vi "simulated camera.vi"(8 "error in (no error)":errorcluster) -> (0 "error out":errorcluster)   [LabVIEW 2018]
uses:
  Sim_Ixon_Ultra/Sim_Ixon_Ultra.lvclass
  C:/Users/Denis/Desktop/S4ACS/S4ACS/Sim_CCD/Sim_CCD.lvclass
  <vilib>/Utility/miscctls.llb/LVDateTimeRec.ctl
  Sim_CCD/Sim_CCD.lvclass/Sim_CCD.ctl
  <vilib>/addons/_JKI Toolkits/Caraya/classes/Assert/Assert Equal Value_Variant.vi
  <vilib>/addons/_JKI Toolkits/Caraya/classes/Assert/Assert Not Error.vi
  <vilib>/addons/_JKI Toolkits/Caraya/classes/Assert/Assert Almost Equal_Float.vi
  <vilib>/addons/_JKI Toolkits/Caraya/classes/Test/Test.lvclass
  <vilib>/addons/_JKI Toolkits/Caraya/classes/Assert/Assert.lvclass
  Sim_CCD/Sim_CCD.lvclass
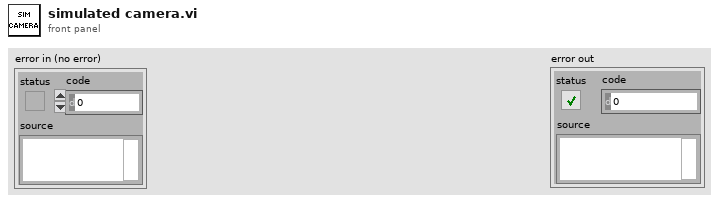
[diagram p1: front panel]
types:
  T1 = cluster{"EXPTIME":dbl, "#FRAMES":u32, "COOLER_POWER_STATUS":u16, "TEMP":i32}
  T2 = cluster{"FRAMES_DONE":u16, "CCD_STATUS":string, "CURRENT_TEMPERATURE":i16, "TEMPERATURE_STATUS":string, "FRAME_EXPOSURE_TIME":sgl, "SERIAL_NUMBER":u16, "ACQUIRING":bool, "POWER":bool, "ACS MODE":bool}
  T3 = cluster{"EXPTIME":errorcluster, "#FRAMES":errorcluster, "COOLER_POWER_STATUS":errorcluster, "TEMP":errorcluster}
  T4 = cluster{"EM_MODE":u16, "EM_GAIN":u16, "FRAME_TRANSFER":bool}
  T5 = cluster{"PREAMP":u16, "READOUT_RATE":u16, "VERTICAL_SHIFT_SPEED":u16, "READ_MODE":u16, "VERTICAL_CLOCK_VOLTAGE":u16, "ACQUISITION_MODE":u16, "AD_CHANNEL":u16, "SHUTTER_TTL":u16, "SHUTTER_OPENING_TIME":u16, "SHUTTER_CLOSING_TIME":u16, "SHUTTER_MODE":u16, "TRIGGER_MODE":u16, "VBIN":u16, "INITIAL_LINE":u16, "INITIAL_COLUMN":u16, "FINAL_LINE":u16, "FINAL_COLUMN":u16, "HBIN":u16}
  T6 = typedef "LVDateTimeRec.ctl" = cluster{"fractional second":dbl, "second":i32, "minute":i32, "hour":i32, "day of month":i32, "month":i32, "year":i32, "day of week":i32, "day of year":i32, "DST":i32}
  T7 = cluster{"Time Acq Started":u32, "Image delay":u64, "Last update - CCD config":timestamp, "SYSTEMTIME":T6, "Readout time":dbl, "Time acq finished":u32, "effective exptime":dbl}
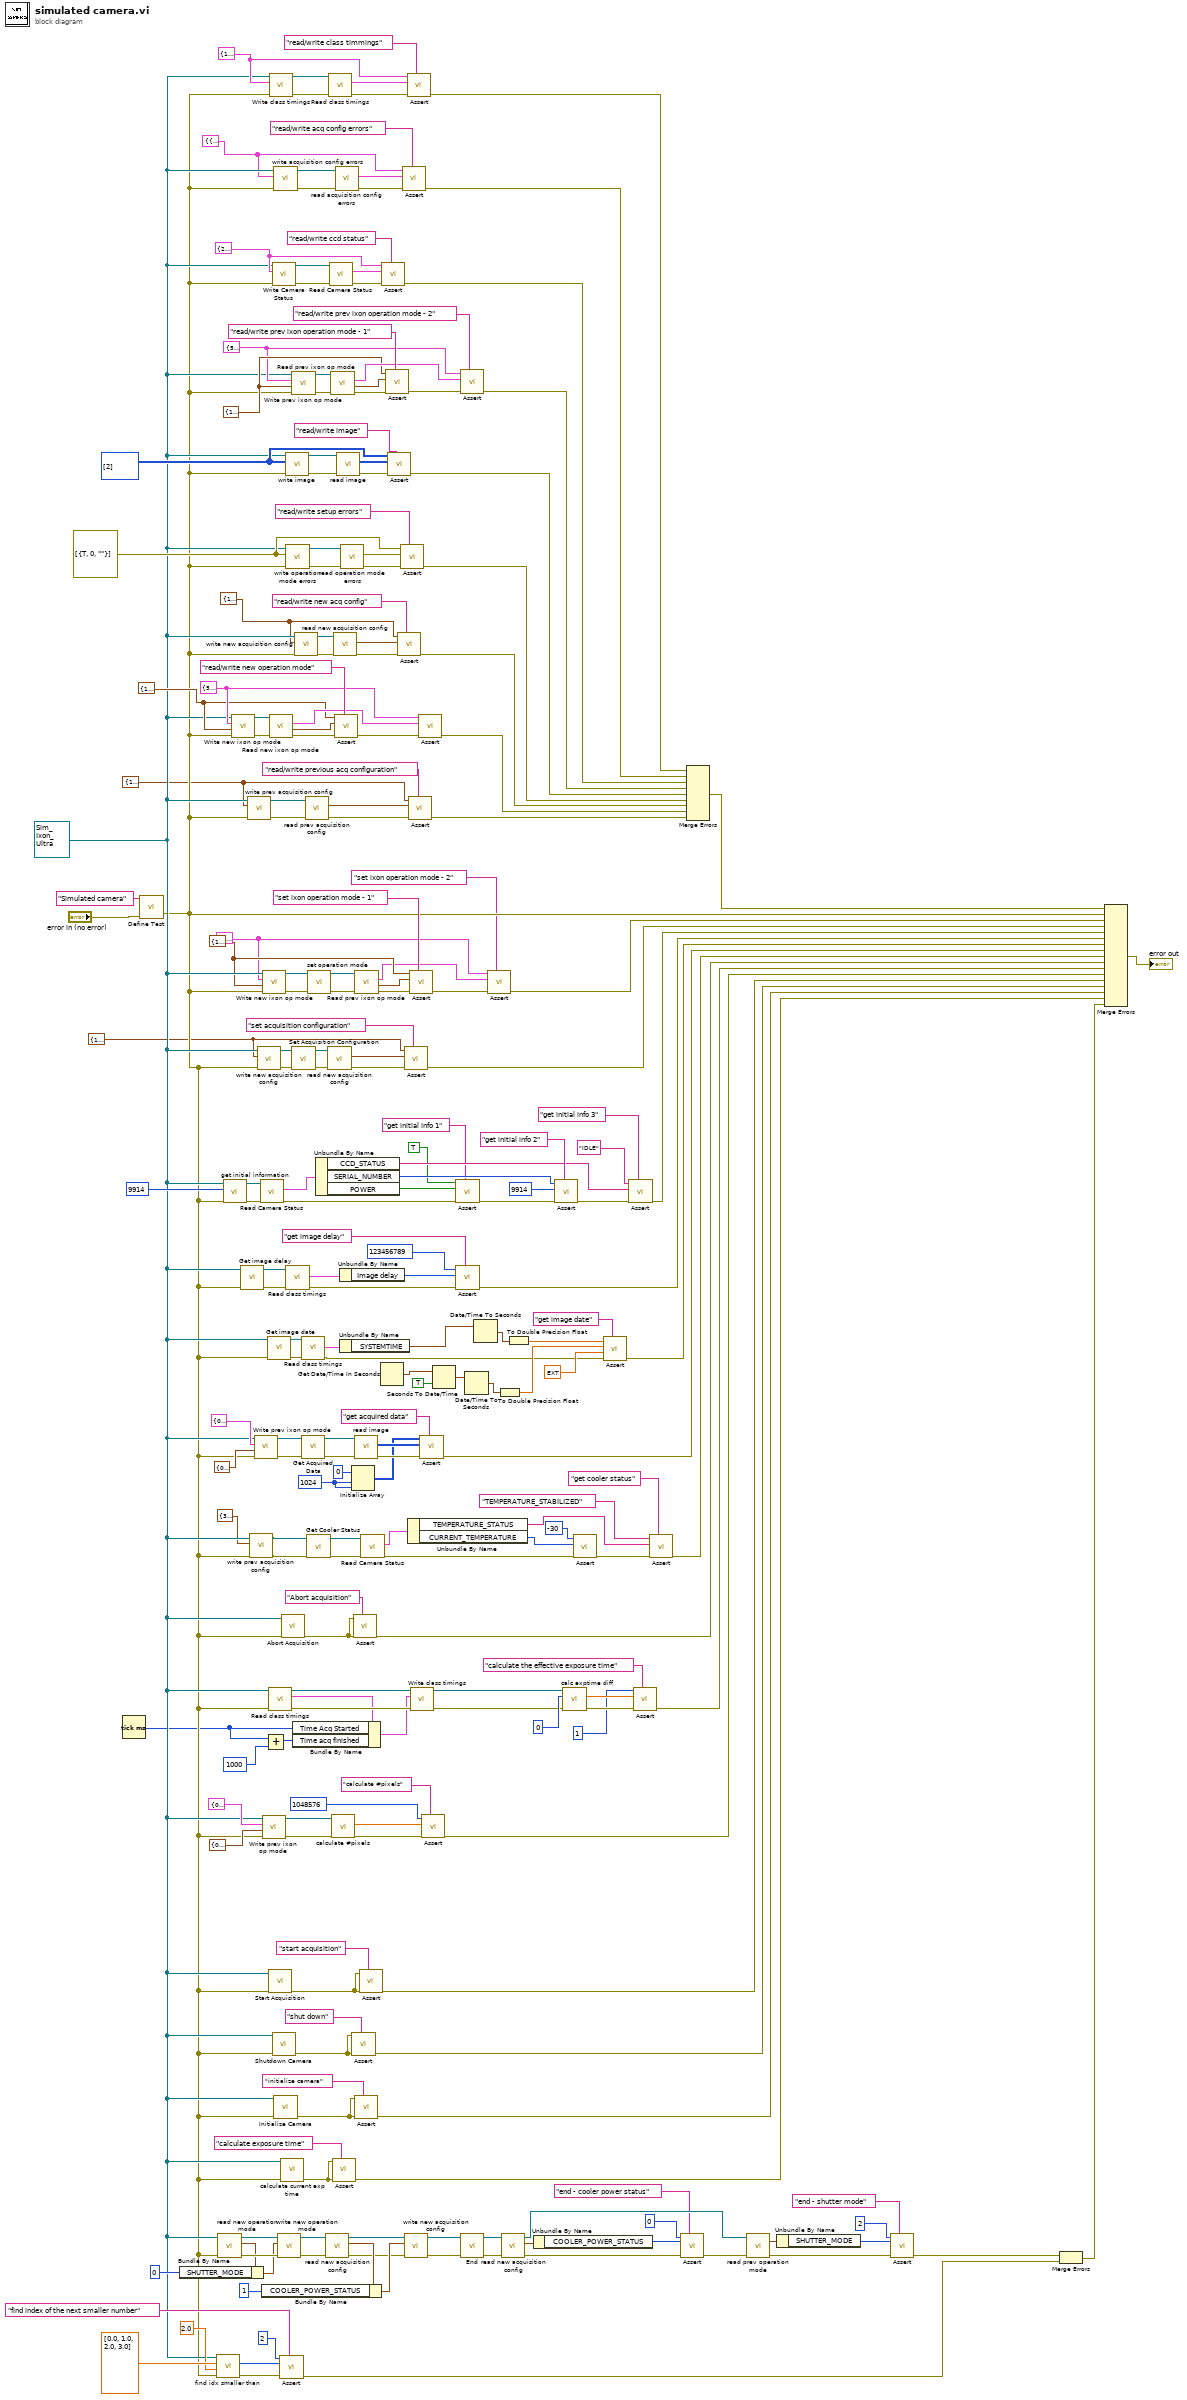
[diagram p0: block diagram]
diagram:
  w85 = T2 {"FRAMES_DONE"=2, "CCD_STATUS"="ASD", "CURRENT_TEMPERATURE"=12, "TEMPERATURE_STATUS"="ABC", "FRAME_EXPOSURE_TIME"=2.0, "SERIAL_NUMBER"=1, "ACQUIRING"=TRUE, "POWER"=TRUE, "ACS MODE"=TRUE} ("camera status")
  w11 = T3 {"EXPTIME"={"status"=TRUE, "code"=4, "source"=""}, "#FRAMES"={"status"=TRUE, "code"=3, "source"=""}, "COOLER_POWER_STATUS"={"status"=TRUE, "code"=2, "source"=""}, "TEMP"={"status"=TRUE, "code"=1, "source"=""}} ("acquisition config errors")
  w12 = T1 {"EXPTIME"=1.0, "#FRAMES"=2, "COOLER_POWER_STATUS"=1, "TEMP"=23} ("prev acquisition configuration")
  w13 = T1 {"EXPTIME"=1.0, "#FRAMES"=2, "COOLER_POWER_STATUS"=1, "TEMP"=23} ("prev acquisition configuration")
  w14 = T1 {"EXPTIME"=1.0, "#FRAMES"=2, "COOLER_POWER_STATUS"=1, "TEMP"=23} ("prev acquisition configuration")
  w16 = T4 {"EM_MODE"=5, "EM_GAIN"=3, "FRAME_TRANSFER"=TRUE} ("prev ixon op mode")
  w18 = T5 {"PREAMP"=1, "READOUT_RATE"=2, "VERTICAL_SHIFT_SPEED"=3, "READ_MODE"=4, "VERTICAL_CLOCK_VOLTAGE"=5, "ACQUISITION_MODE"=6, "AD_CHANNEL"=7, "SHUTTER_TTL"=8, "SHUTTER_OPENING_TIME"=9, "SHUTTER_CLOSING_TIME"=11, "SHUTTER_MODE"=12, "TRIGGER_MODE"=13, "VBIN"=14, "INITIAL_LINE"=15, "INITIAL_COLUMN"=16, "FINAL_LINE"=17, "FINAL_COLUMN"=18, "HBIN"=19} ("prev operation mode")
  w63 = T4 {"EM_MODE"=5, "EM_GAIN"=3, "FRAME_TRANSFER"=TRUE} ("prev ixon op mode")
  w62 = T5 {"PREAMP"=1, "READOUT_RATE"=2, "VERTICAL_SHIFT_SPEED"=3, "READ_MODE"=4, "VERTICAL_CLOCK_VOLTAGE"=5, "ACQUISITION_MODE"=6, "AD_CHANNEL"=7, "SHUTTER_TTL"=8, "SHUTTER_OPENING_TIME"=9, "SHUTTER_CLOSING_TIME"=11, "SHUTTER_MODE"=12, "TRIGGER_MODE"=13, "VBIN"=14, "INITIAL_LINE"=15, "INITIAL_COLUMN"=16, "FINAL_LINE"=17, "FINAL_COLUMN"=18, "HBIN"=19} ("prev operation mode")
  w75 = T4 {"EM_MODE"=5, "EM_GAIN"=3, "FRAME_TRANSFER"=TRUE} ("prev ixon op mode")
  w76 = T5 {"PREAMP"=1, "READOUT_RATE"=2, "VERTICAL_SHIFT_SPEED"=3, "READ_MODE"=4, "VERTICAL_CLOCK_VOLTAGE"=5, "ACQUISITION_MODE"=6, "AD_CHANNEL"=7, "SHUTTER_TTL"=8, "SHUTTER_OPENING_TIME"=9, "SHUTTER_CLOSING_TIME"=11, "SHUTTER_MODE"=12, "TRIGGER_MODE"=13, "VBIN"=14, "INITIAL_LINE"=15, "INITIAL_COLUMN"=16, "FINAL_LINE"=17, "FINAL_COLUMN"=18, "HBIN"=19} ("prev operation mode")
  w90 = T7 {"Time Acq Started"=1, "Image delay"=2, "Last update - CCD config"=timestamp(0 s since 1904-01-01), "SYSTEMTIME"={"fractional second"=3.0, "second"=4, "minute"=5, "hour"=3, "day of month"=7, "month"=8, "year"=5, "day of week"=4, "day of year"=9, "DST"=6}, "Readout time"=0.0, "Time acq finished"=0, "effective exptime"=0.0} ("class timings")
  w31 = refnum<class "Sim_Ixon_Ultra.lvclass"> refnum ("Sim_Ixon_Ultra.lvclass")
  w177 = 1024 ("dimension size")
  w221 = u16[][] [[2]] ("Image Graph")
  w227 = errorcluster[] [{"status"=TRUE, "code"=0, "source"=""}] ("WRITE SETUP errors")
  n1 = Tick Count (ms)() -> (millisecond timer value=w22:u32)
  n2 = call <vilib>:"Define Test.vi"("error in (no error)"="error in (no error)", "Label (VI Title)"="Simulated camera") -> ("error out"=w30:errorcluster)  [unwired: 8 in, 1 out]
  n3 = call "find idx smaller than.vi"("error in (no error)"=w30, "Numeric"=2.0, "Array"=dbl[] [0.0, 1.0, 2.0, 3.0], "Simulated Camera in"=w31) -> ("error out"=w113:errorcluster, "index"=w112:i32)  [unwired: 5 in, 1 out]
  n4 = call "read new operation mode.vi"("error in (no error)"=w30, "CCDCamera in"=w31) -> ("error out"=w132:errorcluster, "new operation mode"=w116:T5, "CCDCamera out"=w133:refnum<class "Sim_Ixon_Ultra.lvclass">)  [unwired: 7 in]
  n5 = Bundle By Name(cluster=w116, "SHUTTER_MODE"=u16 0 ("COOLER_POWER_STATUS")) -> (w131:T5)
  n6 = call-dynamic "get initial information.vi"("error in (no error)"=w30, "SERN"=u16 9914 ("channel"), "Simulated_CCD_Camera in"=w31) -> ("error out"=w205:errorcluster, "Simulated_CCD_Camera out"=w204:refnum<class "Sim_Ixon_Ultra.lvclass">)  [unwired: 7 in]
  n7 = call-dynamic "Write new ixon op mode.vi"("error in (no error)"=w30, "new operation mode"=w62, "new ixon op mode"=w63, "Sim_Ixon_Ultra in"=w31) -> ("error out"=w69:errorcluster, "Sim_Ixon_Ultra out"=w68:refnum<class "Sim_Ixon_Ultra.lvclass">)  [unwired: 6 in]
  n8 = call-dynamic "Get image delay.vi"("error in (no error)"=w30, "Simulated_CCD_Camera in"=w31) -> ("error out"=w52:errorcluster, "Simulated_CCD_Camera out"=w51:refnum<class "Sim_Ixon_Ultra.lvclass">)  [unwired: 8 in]
  n9 = call "write prev acquisition config.vi"("error in (no error)"=w30, "prev acquisition configuration"=w14, "Simulated_CCD_Camera in"=w31) -> ("error out"=w60:errorcluster, "Simulated_CCD_Camera out"=w59:refnum<class "Sim_Ixon_Ultra.lvclass">)  [unwired: 7 in]
  n10 = call "write prev acquisition config.vi"("error in (no error)"=w30, "prev acquisition configuration"=T1 {"EXPTIME"=3.0, "#FRAMES"=4, "COOLER_POWER_STATUS"=1, "TEMP"=-30}, "Simulated_CCD_Camera in"=w31) -> ("error out"=w100:errorcluster, "Simulated_CCD_Camera out"=w101:refnum<class "Sim_Ixon_Ultra.lvclass">)  [unwired: 7 in]
  n11 = call-dynamic "Write prev ixon op mode.vi"("error in (no error)"=w30, "prev operation mode"=T5 {"PREAMP"=0, "READOUT_RATE"=0, "VERTICAL_SHIFT_SPEED"=0, "READ_MODE"=0, "VERTICAL_CLOCK_VOLTAGE"=0, "ACQUISITION_MODE"=0, "AD_CHANNEL"=0, "SHUTTER_TTL"=0, "SHUTTER_OPENING_TIME"=0, "SHUTTER_CLOSING_TIME"=0, "SHUTTER_MODE"=0, "TRIGGER_MODE"=0, "VBIN"=1, "INITIAL_LINE"=1, "INITIAL_COLUMN"=1, "FINAL_LINE"=1024, "FINAL_COLUMN"=1024, "HBIN"=1}, "prev ixon op mode"=T4 {"EM_MODE"=0, "EM_GAIN"=2, "FRAME_TRANSFER"=FALSE}, "Sim_Ixon_Ultra in"=w31) -> ("error out"=w99:errorcluster, "Sim_Ixon_Ultra out"=w98:refnum<class "Sim_Ixon_Ultra.lvclass">)  [unwired: 6 in]
  n12 = call "write new acquisition config.vi"("error in (no error)"=w30, "new acquisition configuration"=w13, "Simulated_CCD_Camera in"=w31) -> ("error out"=w47:errorcluster, "Simulated_CCD_Camera out"=w46:refnum<class "Sim_Ixon_Ultra.lvclass">)  [unwired: 7 in]
  n13 = call "Read Camera Status.vi"("error in (no error)"=w205, "CCDCamera in"=w204) -> ("error out"=w41:errorcluster, "camera status"=w203:T2)  [unwired: 7 in, 1 out]
  n14 = call-dynamic "Write prev ixon op mode.vi"("error in (no error)"=w30, "prev operation mode"=T5 {"PREAMP"=0, "READOUT_RATE"=0, "VERTICAL_SHIFT_SPEED"=0, "READ_MODE"=0, "VERTICAL_CLOCK_VOLTAGE"=0, "ACQUISITION_MODE"=0, "AD_CHANNEL"=0, "SHUTTER_TTL"=0, "SHUTTER_OPENING_TIME"=0, "SHUTTER_CLOSING_TIME"=0, "SHUTTER_MODE"=0, "TRIGGER_MODE"=0, "VBIN"=1, "INITIAL_LINE"=1, "INITIAL_COLUMN"=1, "FINAL_LINE"=1024, "FINAL_COLUMN"=1024, "HBIN"=1}, "prev ixon op mode"=T4 {"EM_MODE"=0, "EM_GAIN"=2, "FRAME_TRANSFER"=FALSE}, "Sim_Ixon_Ultra in"=w31) -> ("error out"=w104:errorcluster, "Sim_Ixon_Ultra out"=w103:refnum<class "Sim_Ixon_Ultra.lvclass">)  [unwired: 6 in]
  n15 = call-dynamic "Write new ixon op mode.vi"("error in (no error)"=w30, "new operation mode"=w18, "new ixon op mode"=w16, "Sim_Ixon_Ultra in"=w31) -> ("error out"=w53:errorcluster, "Sim_Ixon_Ultra out"=w54:refnum<class "Sim_Ixon_Ultra.lvclass">)  [unwired: 6 in]
  n16 = Add(x=w22, y=u32 1000) -> (x+y=w23:u32)
  n17 = call-dynamic "Get image date.vi"("error in (no error)"=w30, "Simulated_CCD_Camera in"=w31) -> ("error out"=w35:errorcluster, "Simulated_CCD_Camera out"=w36:refnum<class "Sim_Ixon_Ultra.lvclass">)  [unwired: 8 in]
  n18 = call "Read class timings.vi"("error in (no error)"=w30, "Simulated Camera in"=w31) -> ("error out"=w26:errorcluster, "class timings"=w25:T7, "Simulated Camera out"=w29:refnum<class "Sim_Ixon_Ultra.lvclass">)  [unwired: 7 in]
  n19 = call-dynamic "Start Acquisition.vi"("error in (no error)"=w30, "CCDCamera in"=w31) -> ("error out"=w144:errorcluster)  [unwired: 8 in, 1 out]
  n20 = call "Write class timings.vi"("error in (no error)"=w30, "class timings"=w90, "Simulated Camera in"=w31) -> ("error out"=w92:errorcluster, "Simulated Camera out"=w93:refnum<class "Sim_Ixon_Ultra.lvclass">)  [unwired: 7 in]
  n21 = call-dynamic "Read new ixon op mode.vi"("error in (no error)"=w69, "Sim_Ixon_Ultra in"=w68) -> ("error out"=w70:errorcluster, "new operation mode"=w67:T5, "new ixon op mode"=w64:T4)  [unwired: 6 in, 1 out]
  n22 = call "Write Camera Status.vi"("error in (no error)"=w30, "camera status"=w85, "CCDCamera in"=w31) -> ("error out"=w217:errorcluster, "CCDCamera out"=w216:refnum<class "Sim_Ixon_Ultra.lvclass">)  [unwired: 7 in]
  n23 = call-dynamic "Shutdown Camera.vi"("error in (no error)"=w30, "CCDCamera in"=w31) -> ("error out"=w142:errorcluster)  [unwired: 8 in, 1 out]
  n24 = call "write acquisition config errors.vi"("error in (no error)"=w30, "acquisition config errors"=w11, "Simulated Camera in"=w31) -> ("error out"=w86:errorcluster, "Simulated Camera out"=w87:refnum<class "Sim_Ixon_Ultra.lvclass">)  [unwired: 7 in]
  n25 = call-dynamic "Initialize Camera.vi"("error in (no error)"=w30, "CCDCamera in"=w31) -> ("error out"=w140:errorcluster)  [unwired: 8 in, 1 out]
  n26 = call "write new operation mode.vi"("error in (no error)"=w132, "new operation mode"=w131, "CCDCamera in"=w133) -> ("error out"=w10:errorcluster, "CCDCamera out"=w9:refnum<class "Sim_Ixon_Ultra.lvclass">)  [unwired: 7 in]
  n27 = call-poly <vilib>:"Assert.vi"("Label"="find index of the next smaller number" ("format string"), "error in (no error)"=w113, "Actual"=w112, "Expected"=u16 2 ("COOLER_POWER_STATUS")) -> ("error out"=w110:errorcluster)  [unwired: 6 in, 1 out]
  n28 = call-dynamic "calculate current exp time.vi"("error in (no error)"=w30, "CCDCamera in"=w31) -> ("error out"=w105:errorcluster)  [unwired: 8 in, 1 out]
  n29 = call-dynamic "Abort Acquisition.vi"("error in (no error)"=w30, "CCDCamera in"=w31) -> ("error out"=w161:errorcluster)  [unwired: 8 in, 1 out]
  n30 = call "write image.vi"("error in (no error)"=w30, "Image Graph"=w221, "CCDCamera in"=w31) -> ("error out"=w225:errorcluster, "CCDCamera out"=w224:refnum<class "Sim_Ixon_Ultra.lvclass">)  [unwired: 7 in]
  n31 = call "write operation mode errors.vi"("error in (no error)"=w30, "WRITE SETUP errors"=w227, "Simulated_CCD_Camera in"=w31) -> ("error out"=w234:errorcluster, "Simulated_CCD_Camera out"=w233:refnum<class "Sim_Ixon_Ultra.lvclass">)  [unwired: 7 in]
  n32 = call "Read class timings.vi"("error in (no error)"=w52, "Simulated Camera in"=w51) -> ("error out"=w50:errorcluster, "class timings"=w49:T7)  [unwired: 7 in, 1 out]
  n33 = call-dynamic "Write prev ixon op mode.vi"("error in (no error)"=w30, "prev operation mode"=w76, "prev ixon op mode"=w75, "Sim_Ixon_Ultra in"=w31) -> ("error out"=w84:errorcluster, "Sim_Ixon_Ultra out"=w83:refnum<class "Sim_Ixon_Ultra.lvclass">)  [unwired: 6 in]
  n34 = call-dynamic "Set Acquisition Configuration.vi"("error in (no error)"=w47, "CCDCamera in"=w46) -> ("error out"=w45:errorcluster, "CCDCamera out"=w44:refnum<class "Sim_Ixon_Ultra.lvclass">)  [unwired: 8 in]
  n35 = Bundle By Name(cluster=w25, "Time Acq Started"=w22, "Time acq finished"=w23) -> (w24:T7)
  n36 = call "write new acquisition config.vi"("error in (no error)"=w30, "new acquisition configuration"=w12, "Simulated_CCD_Camera in"=w31) -> ("error out"=w72:errorcluster, "Simulated_CCD_Camera out"=w71:refnum<class "Sim_Ixon_Ultra.lvclass">)  [unwired: 7 in]
  n37 = call "Read class timings.vi"("error in (no error)"=w35, "Simulated Camera in"=w36) -> ("error out"=w32:errorcluster, "class timings"=w34:T7)  [unwired: 7 in, 1 out]
  n38 = call-dynamic "Get Acquired Data.vi"("error in (no error)"=w99, "CCDCamera in"=w98) -> ("error out"=w180:errorcluster, "CCDCamera out"=w181:refnum<class "Sim_Ixon_Ultra.lvclass">)  [unwired: 8 in]
  n39 = call "read prev acquisition config.vi"("error in (no error)"=w60, "Simulated_CCD_Camera in"=w59) -> ("error out"=w61:errorcluster, "prev acquisition configuration"=w58:T1)  [unwired: 7 in, 1 out]
  n40 = call-dynamic "Get Cooler Status.vi"("error in (no error)"=w100, "CCDCamera in"=w101) -> ("error out"=w171:errorcluster, "CCDCamera out"=w172:refnum<class "Sim_Ixon_Ultra.lvclass">)  [unwired: 8 in]
  n41 = call-dynamic "set operation mode.vi"("error in (no error)"=w53, "CCDCamera in"=w54) -> ("error out"=w55:errorcluster, "CCDCamera out"=w56:refnum<class "Sim_Ixon_Ultra.lvclass">)  [unwired: 8 in]
  n42 = Unbundle By Name(w203) -> ("CCD_STATUS"=w198:string, "SERIAL_NUMBER"=w202:u16, "POWER"=w39:bool)
  n43 = call "read new acquisition config.vi"("error in (no error)"=w10, "Simulated_CCD_Camera in"=w9) -> ("error out"=w4:errorcluster, "new acquisition configuration"=w6:T1, "Simulated_CCD_Camera out"=w3:refnum<class "Sim_Ixon_Ultra.lvclass">)  [unwired: 7 in]
  n44 = Bundle By Name(cluster=w6, "COOLER_POWER_STATUS"=u16 1) -> (w5:T1)
  n45 = call "read new acquisition config.vi"("error in (no error)"=w45, "Simulated_CCD_Camera in"=w44) -> ("error out"=w43:errorcluster, "new acquisition configuration"=w42:T1)  [unwired: 7 in, 1 out]
  n46 = call "Read class timings.vi"("error in (no error)"=w92, "Simulated Camera in"=w93) -> ("error out"=w94:errorcluster, "class timings"=w91:T7)  [unwired: 7 in, 1 out]
  n47 = call "Read Camera Status.vi"("error in (no error)"=w217, "CCDCamera in"=w216) -> ("error out"=w215:errorcluster, "camera status"=w213:T2)  [unwired: 7 in, 1 out]
  n48 = call-dynamic "Read prev ixon op mode.vi"("error in (no error)"=w84, "Sim_Ixon_Ultra in"=w83) -> ("error out"=w82:errorcluster, "prev operation mode"=w81:T5, "prev ixon op mode"=w78:T4)  [unwired: 6 in, 1 out]
  n49 = call "calculate #pixels.vi"("error in (no error)"=w104, "Simulated Camera in"=w103) -> ("error out"=w149:errorcluster, "#pixels"=w148:dbl)  [unwired: 7 in, 1 out]
  n50 = call-poly <vilib>:"Assert.vi"("Label"="calculate exposure time" ("format string"), "error in (no error)"=w105, "Not Error?"=w105) -> ("error out"=w134:errorcluster)  [unwired: 7 in, 1 out]
  n51 = call "read new acquisition config.vi"("error in (no error)"=w72, "Simulated_CCD_Camera in"=w71) -> ("error out"=w74:errorcluster, "new acquisition configuration"=w73:T1)  [unwired: 7 in, 1 out]
  n52 = call-poly <vilib>:"Assert.vi"("Label"="read/write new operation mode", "error in (no error)"=w70, "Actual"=w67, "Expected"=w62) -> ("error out"=w66:errorcluster)  [unwired: 6 in, 1 out]
  n53 = call "read acquisition config errors.vi"("error in (no error)"=w86, "Simulated Camera in"=w87) -> ("error out"=w89:errorcluster, "acquisition config errors"=w88:T3)  [unwired: 7 in, 1 out]
  n54 = call "read image.vi"("error in (no error)"=w225, "CCDCamera in"=w224) -> ("error out"=w223:errorcluster, "Image Graph"=w222:u16[][])  [unwired: 7 in, 1 out]
  n55 = Unbundle By Name(w49) -> ("Image delay"=w48:u64)
  n56 = Unbundle By Name(w34) -> ("SYSTEMTIME"=w33:T6)
  n57 = call "read operation mode errors.vi"("error in (no error)"=w234, "Simulated_CCD_Camera in"=w233) -> ("error out"=w230:errorcluster, "WRITE SETUP errors"=w228:errorcluster[])  [unwired: 7 in, 1 out]
  n58 = Initialize Array(u16 0, w177, w177) -> (w175:u16[][])
  n59 = call-poly <vilib>:"Assert.vi"("Label"="shut down" ("format string"), "error in (no error)"=w142, "Not Error?"=w142) -> ("error out"=w137:errorcluster)  [unwired: 7 in, 1 out]
  n60 = call-poly <vilib>:"Assert.vi"("Label"="Abort acquisition" ("Label (VI Title)"), "error in (no error)"=w161, "Not Error?"=w161) -> ("error out"=w159:errorcluster)  [unwired: 7 in, 1 out]
  n61 = call "read image.vi"("error in (no error)"=w180, "CCDCamera in"=w181) -> ("error out"=w178:errorcluster, "Image Graph"=w176:u16[][])  [unwired: 7 in, 1 out]
  n62 = call-poly <vilib>:"Assert.vi"("Label"="initialize camera" ("format string"), "error in (no error)"=w140, "Not Error?"=w140) -> ("error out"=w136:errorcluster)  [unwired: 7 in, 1 out]
  n63 = call-dynamic "Read prev ixon op mode.vi"("error in (no error)"=w55, "Sim_Ixon_Ultra in"=w56) -> ("error out"=w57:errorcluster, "prev operation mode"=w19:T5, "prev ixon op mode"=w17:T4)  [unwired: 6 in, 1 out]
  n64 = call-poly <vilib>:"Assert.vi"("Label"="start acquisition" ("format string"), "error in (no error)"=w144, "Not Error?"=w144) -> ("error out"=w138:errorcluster)  [unwired: 7 in, 1 out]
  n65 = call "Read Camera Status.vi"("error in (no error)"=w171, "CCDCamera in"=w172) -> ("error out"=w170:errorcluster, "camera status"=w169:T2)  [unwired: 7 in, 1 out]
  n66 = Get Date/Time In Seconds() -> (seconds since 1Jan1904=w190:timestamp)
  n67 = call-poly <vilib>:"Assert.vi"("Label"="read/write ccd status", "error in (no error)"=w215, "Actual"=w213, "Expected"=w85) -> ("error out"=w214:errorcluster)  [unwired: 6 in, 1 out]
  n68 = call-poly <vilib>:"Assert.vi"("Label"="read/write prev ixon operation mode - 1", "error in (no error)"=w82, "Actual"=w81, "Expected"=w76) -> ("error out"=w80:errorcluster)  [unwired: 6 in, 1 out]
  n69 = call-poly <vilib>:"Assert.vi"("Label"="read/write image", "error in (no error)"=w223, "Actual"=w222, "Expected"=w221) -> ("error out"=w219:errorcluster)  [unwired: 6 in, 1 out]
  n70 = call-poly <vilib>:"Assert.vi"("Label"="read/write new acq config", "error in (no error)"=w74, "Actual"=w73, "Expected"=w12) -> ("error out"=w235:errorcluster)  [unwired: 6 in, 1 out]
  n71 = call-poly <vilib>:"Assert.vi"("Label"="read/write setup errors", "error in (no error)"=w230, "Actual"=w228, "Expected"=w227) -> ("error out"=w229:errorcluster)  [unwired: 6 in, 1 out]
  n72 = call-poly <vilib>:"Assert.vi"("Label"="read/write acq config errors", "error in (no error)"=w89, "Actual"=w88, "Expected"=w11) -> ("error out"=w210:errorcluster)  [unwired: 6 in, 1 out]
  n73 = call-poly <vilib>:"Assert.vi"("Label"="set acquisition configuration" ("Label (VI Title)"), "error in (no error)"=w43, "Actual"=w42, "Expected"=w13) -> ("error out"=w209:errorcluster)  [unwired: 6 in, 1 out]
  n74 = call "write new acquisition config.vi"("error in (no error)"=w4, "new acquisition configuration"=w5, "Simulated_CCD_Camera in"=w3) -> ("error out"=w7:errorcluster, "Simulated_CCD_Camera out"=w8:refnum<class "Sim_Ixon_Ultra.lvclass">)  [unwired: 7 in]
  n75 = call-poly <vilib>:"Assert.vi"("Label"="read/write class timmings", "error in (no error)"=w94, "Actual"=w91, "Expected"=w90) -> ("error out"=w155:errorcluster)  [unwired: 6 in, 1 out]
  n76 = Unbundle By Name(w169) -> ("TEMPERATURE_STATUS"=w165:string, "CURRENT_TEMPERATURE"=w168:i16)
  n77 = call-poly <vilib>:"Assert.vi"("Label"="read/write previous acq configuration", "error in (no error)"=w61, "Actual"=w58, "Expected"=w14) -> ("error out"=w236:errorcluster)  [unwired: 6 in, 1 out]
  n78 = call-poly <vilib>:"Assert.vi"("Label"="set ixon operation mode - 1" ("Label (VI Title)"), "error in (no error)"=w57, "Actual"=w19, "Expected"=w18) -> ("error out"=w21:errorcluster)  [unwired: 6 in, 1 out]
  n79 = call "Write class timings.vi"("error in (no error)"=w26, "class timings"=w24, "Simulated Camera in"=w29) -> ("error out"=w27:errorcluster, "Simulated Camera out"=w28:refnum<class "Sim_Ixon_Ultra.lvclass">)  [unwired: 7 in]
  n80 = call-poly <vilib>:"Assert.vi"("error in (no error)"=w66, "Actual"=w64, "Expected"=w63) -> ("error out"=w65:errorcluster)  [unwired: 7 in, 1 out]
  n81 = call-poly <vilib>:"Assert.vi"("Label"="get acquired data" ("Label (VI Title)"), "error in (no error)"=w178, "Actual"=w176, "Expected"=w175) -> ("error out"=w174:errorcluster)  [unwired: 6 in, 1 out]
  n82 = call-poly <vilib>:"Assert.vi"("Label"="calculate #pixels" ("Label (VI Title)"), "error in (no error)"=w149, "Actual"=w148, "Expected"=u32 1048576 ("y")) -> ("error out"=w145:errorcluster)  [unwired: 6 in, 1 out]
  n83 = Seconds To Date/Time(time stamp (now)=w190, to UTC (F)=TRUE) -> (date time rec=w189:T6)
  n84 = call-poly <vilib>:"Assert.vi"("Label"="get initial info 1" ("Label (VI Title)"), "error in (no error)"=w41, "Actual"=w39, "Expected"=TRUE) -> ("error out"=w40:errorcluster)  [unwired: 6 in, 1 out]
  n85 = call-poly <vilib>:"Assert.vi"("Label"="get image delay" ("Label (VI Title)"), "error in (no error)"=w50, "Actual"=w48, "Expected"=u32 123456789 ("channel")) -> ("error out"=w192:errorcluster)  [unwired: 6 in, 1 out]
  n86 = call-poly <vilib>:"Assert.vi"("Label"="read/write prev ixon operation mode - 2", "error in (no error)"=w80, "Actual"=w78, "Expected"=w75) -> ("error out"=w79:errorcluster)  [unwired: 6 in, 1 out]
  n87 = call "End.vi"("error in (no error)"=w7, "Simulated_CCD_Camera in"=w8) -> ("error out"=w130:errorcluster, "Simulated_CCD_Camera out"=w129:refnum<class "Sim_Ixon_Ultra.lvclass">)  [unwired: 8 in]
  n88 = Date/Time To Seconds(2:w189) -> (0:w188:timestamp)  [unwired: 1 in]
  n89 = Date/Time To Seconds(2:w33) -> (0:w187:timestamp)  [unwired: 1 in]
  n90 = call-poly <vilib>:"Assert.vi"("Label"="set ixon operation mode - 2" ("Label (VI Title)"), "error in (no error)"=w21, "Actual"=w17, "Expected"=w16) -> ("error out"=w20:errorcluster)  [unwired: 6 in, 1 out]
  n91 = To Double Precision Float(number=w188) -> (double precision float=w185:dbl)
  n92 = call "read new acquisition config.vi"("error in (no error)"=w130, "Simulated_CCD_Camera in"=w129) -> ("error out"=w128:errorcluster, "new acquisition configuration"=w127:T1, "Simulated_CCD_Camera out"=w123:refnum<class "Sim_Ixon_Ultra.lvclass">)  [unwired: 7 in]
  n93 = To Double Precision Float(number=w187) -> (double precision float=w186:dbl)
  n94 = Unbundle By Name(w127) -> ("COOLER_POWER_STATUS"=w126:u16)
  n95 = call-poly <vilib>:"Assert.vi"("Label"="get initial info 2" ("Label (VI Title)"), "error in (no error)"=w40, "Actual"=u16 9914 ("channel"), "Expected"=w202) -> ("error out"=w199:errorcluster)  [unwired: 6 in, 1 out]
  n96 = call-dynamic "calc exptime diff.vi"("error in (no error)"=w27, "ACS mode"=0, "Simulated_CCD_Camera in"=w28) -> ("error out"=w153:errorcluster, "effective exptime"=w152:dbl)  [unwired: 6 in, 1 out]
  n97 = call-poly <vilib>:"Assert.vi"("error in (no error)"=w170, "Actual"=w168, "Expected"=-30 ("dimension size")) -> ("error out"=w166:errorcluster)  [unwired: 7 in, 1 out]
  n98 = call-poly <vilib>:"Assert.vi"("Label"="get image date" ("Label (VI Title)"), "error in (no error)"=w32, "Tolerance"=ext 0.1, "Actual"=w185, "Expected"=w186) -> ("error out"=w183:errorcluster)  [unwired: 5 in, 1 out]
  n99 = call-poly <vilib>:"Assert.vi"("Label"="get initial info 3" ("Label (VI Title)"), "error in (no error)"=w199, "Actual"=w198, "Expected"="IDLE" ("Label (VI Title)")) -> ("error out"=w195:errorcluster)  [unwired: 6 in, 1 out]
  n100 = call-poly <vilib>:"Assert.vi"("Label"="calculate the effective exposure time" ("Label (VI Title)"), "error in (no error)"=w153, "Actual"=w152, "Expected"=u32 1 ("y")) -> ("error out"=w154:errorcluster)  [unwired: 6 in, 1 out]
  n101 = call-poly <vilib>:"Assert.vi"("Label"="get cooler status" ("Label (VI Title)"), "error in (no error)"=w166, "Actual"=w165, "Expected"="TEMPERATURE_STABILIZED" ("Label (VI Title)")) -> ("error out"=w162:errorcluster)  [unwired: 6 in, 1 out]
  n102 = call-poly <vilib>:"Assert.vi"("Label"="end - cooler power status" ("format string"), "error in (no error)"=w128, "Actual"=w126, "Expected"=u16 0 ("SHUTTER_MODE")) -> ("error out"=w124:errorcluster)  [unwired: 6 in, 1 out]
  n103 = Merge Errors(w155, w210, w214, w79, w219, w229, w235, w65, w236) -> (w238:errorcluster)
  n104 = call "read prev operation mode.vi"("error in (no error)"=w124, "Simulated_CCD_Camera in"=w123) -> ("error out"=w121:errorcluster, "prev operation mode"=w122:T5)  [unwired: 7 in, 1 out]
  n105 = Unbundle By Name(w122) -> ("SHUTTER_MODE"=w120:u16)
  n106 = call-poly <vilib>:"Assert.vi"("Label"="end - shutter mode" ("format string"), "error in (no error)"=w121, "Actual"=w120, "Expected"=u16 2 ("SHUTTER_MODE")) -> ("error out"=w117:errorcluster)  [unwired: 6 in, 1 out]
  n107 = Merge Errors(w117, w110) -> (w118:errorcluster)
  n108 = Merge Errors(w238, w30, w20, w209, w195, w192, w183, w174, w162, w159, w154, w145, w138, w137, w136, w134, w118) -> (→"error out":errorcluster)
